vi "Unit Test.vi"   [LabVIEW 2019, in "Initialize.lvlib"]
uses:
  Initialize.lvlib
  User Event/Controls/UE Abort Action.ctl
  IO/sbRIO9623/sbRIO9623.lvlib
  Laser/Coherent/Coherent.lvlib
  LED/LED.lvlib
  Motion/Allmotion/Allmotion.lvlib
  Selection Valve/IDEX/IDEX.lvlib
  Syringe Pump/NE-500/NE-500.lvlib
  Fluidic Process/Fluidic Process.lvlib
  Image/Image.lvlib
  Camera/Andor/Andor.lvlib
types:
  T1 = typedef "UE Abort Action.ctl" = enum16{"Create", "Get", "Destroy"}
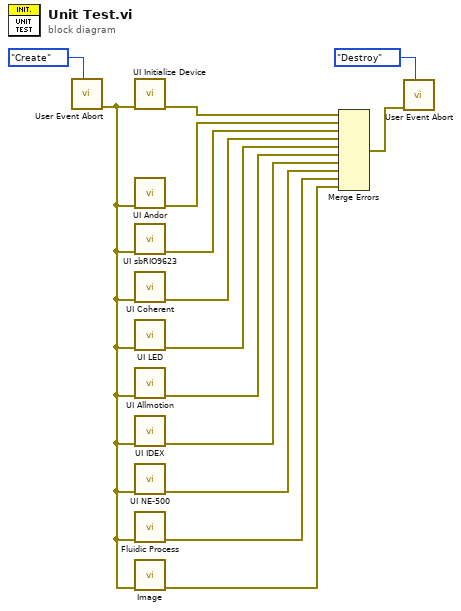
[diagram p0: block diagram]
diagram:
  n1 = call "User Event Abort.vi"("Action"=UE_Abort_Action."Create") -> ("Error Out"=w3:errorcluster)  [unwired: 9 in, 1 out]
  n2 = call "UI Initialize Device.vi"("error in"=w3) -> ("error out"=w2:errorcluster)  [unwired: 10 in]
  n3 = call "UI Andor.vi"("error in"=w3) -> ("error out"=w1:errorcluster)  [unwired: 10 in]
  n4 = call "UI sbRIO9623.vi"("error in"=w3) -> ("error out"=w11:errorcluster)  [unwired: 10 in]
  n5 = call "UI Coherent.vi"("error in"=w3) -> ("error out"=w10:errorcluster)  [unwired: 10 in]
  n6 = call "UI LED.vi"("error in"=w3) -> ("error out"=w9:errorcluster)  [unwired: 10 in]
  n7 = call "UI Allmotion.vi"("error in"=w3) -> ("error out"=w8:errorcluster)  [unwired: 10 in]
  n8 = call "UI IDEX.vi"("error in"=w3) -> ("error out"=w7:errorcluster)  [unwired: 10 in]
  n9 = call "UI NE-500.vi"("error in"=w3) -> ("error out"=w6:errorcluster)  [unwired: 10 in]
  n10 = call "Fluidic Process.vi"("error in"=w3) -> ("error out"=w5:errorcluster)  [unwired: 10 in]
  n11 = call "Image.vi"("error in"=w3) -> ("error out"=w4:errorcluster)  [unwired: 10 in]
  n12 = Merge Errors(w2, w1, w11, w10, w9, w8, w7, w6, w5, w4) -> (w12:errorcluster)
  n13 = call "User Event Abort.vi"("Action"=UE_Abort_Action."Destroy", "Error In"=w12) -> ()  [unwired: 8 in, 2 out]
